vi "ref_INT_offset.vi"(10 "ST_reference_info":T1, 11 "INT_position":i16) -> (3 "reference_byte_array_offset":i32)   [LabVIEW 2020]
uses:
  ST_reference_info.ctl
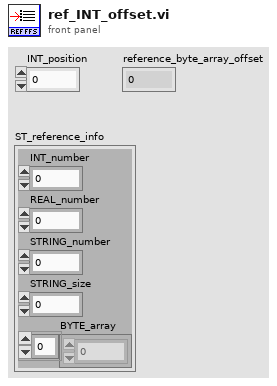
[diagram p1: front panel]
types:
  T1 = typedef "ST_reference_info.ctl" = cluster{"INT_number":i32, "REAL_number":i32, "STRING_number":i32, "STRING_size":i32, "BYTE_array":u8[]}
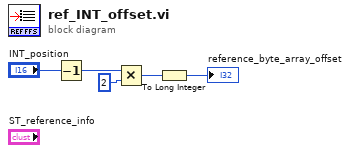
[diagram p0: block diagram]
diagram:
  n1 = Decrement(x="INT_position") -> (x-1=w1:i16)
  n2 = Multiply(x=w1, y=i16 2) -> (x*y=w3:i16)
  n3 = To Long Integer(number=w3) -> (32bit integer=→"reference_byte_array_offset":i32)
